vi "AMI_Extrae_SetField Y.vi"(10 "String":string="Set Y Axis Magnetic Field 0.100Tesla at 0.030Tesla/min, PAUSE, Wait") -> (1 "Array":string[](array[string]))   [LabVIEW 2017]
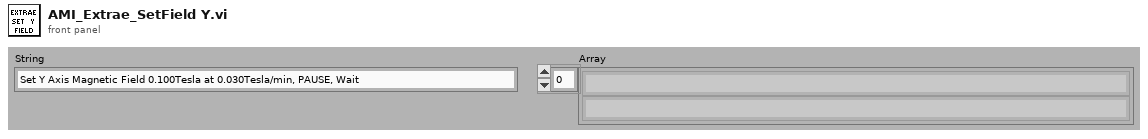
[diagram p1: front panel]
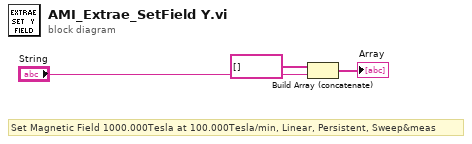
[diagram p0: block diagram]
diagram:
  # "Set Magnetic Field 1000.000Tesla at 100.000Tesla/min, Linear, Persistent, Sweep&meas"
  n1 = Build Array (concatenate)(string[] [] ("Array I"), "String") -> (→"Array":string[])
